vi "subDetermineNeedRebuildingFromHashes.vi"(8 "Force rebuild":bool, 9 "Dependency files":set{path}(c389), 10 "ProjectItem in":refnum<class "ProjectItem.lvclass">, 11 "Hashes in":T1) -> (1 "Needs rebuilding":bool, 2 "Log string":string, 3 "Hashes out":T1)   [LabVIEW 2019, in "SolutionBuilder.lvlib" / "SolutionBuilder.lvclass"]
uses:
  SolutionBuilder.lvclass
  Hashes.ctl
  HashMap.ctl
  IncrementalProjectInfo.ctl
  ProjectItem/ProjectItem.lvclass
  <vilib>/Utility/miscctls.llb/LVMapReplaceAction.ctl
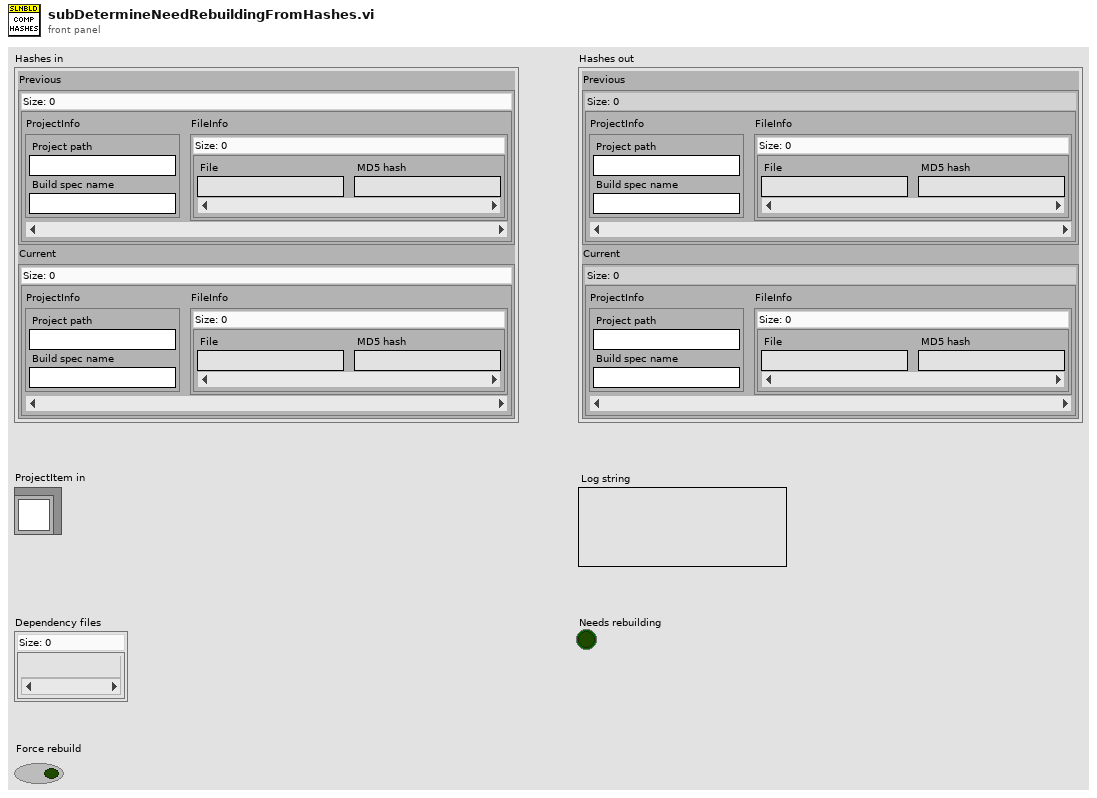
[diagram p1: front panel]
types:
  T1 = typedef "SolutionBuilder.lvlib/SolutionBuilder.lvclass/Hashes.ctl" = cluster{"Previous":T2, "Current":T2}
  T2 = typedef "SolutionBuilder.lvlib/SolutionBuilder.lvclass/HashMap.ctl" = map{T3, map{string, string}}
  T3 = typedef "SolutionBuilder.lvlib/SolutionBuilder.lvclass/IncrementalProjectInfo.ctl" = cluster{"Project path":string, "Build spec name":string}
  T4 = typedef "LVMapReplaceAction.ctl" = enum32{"Modify Entry only if found", "Add or Modify Entry", "Delete Entry"}
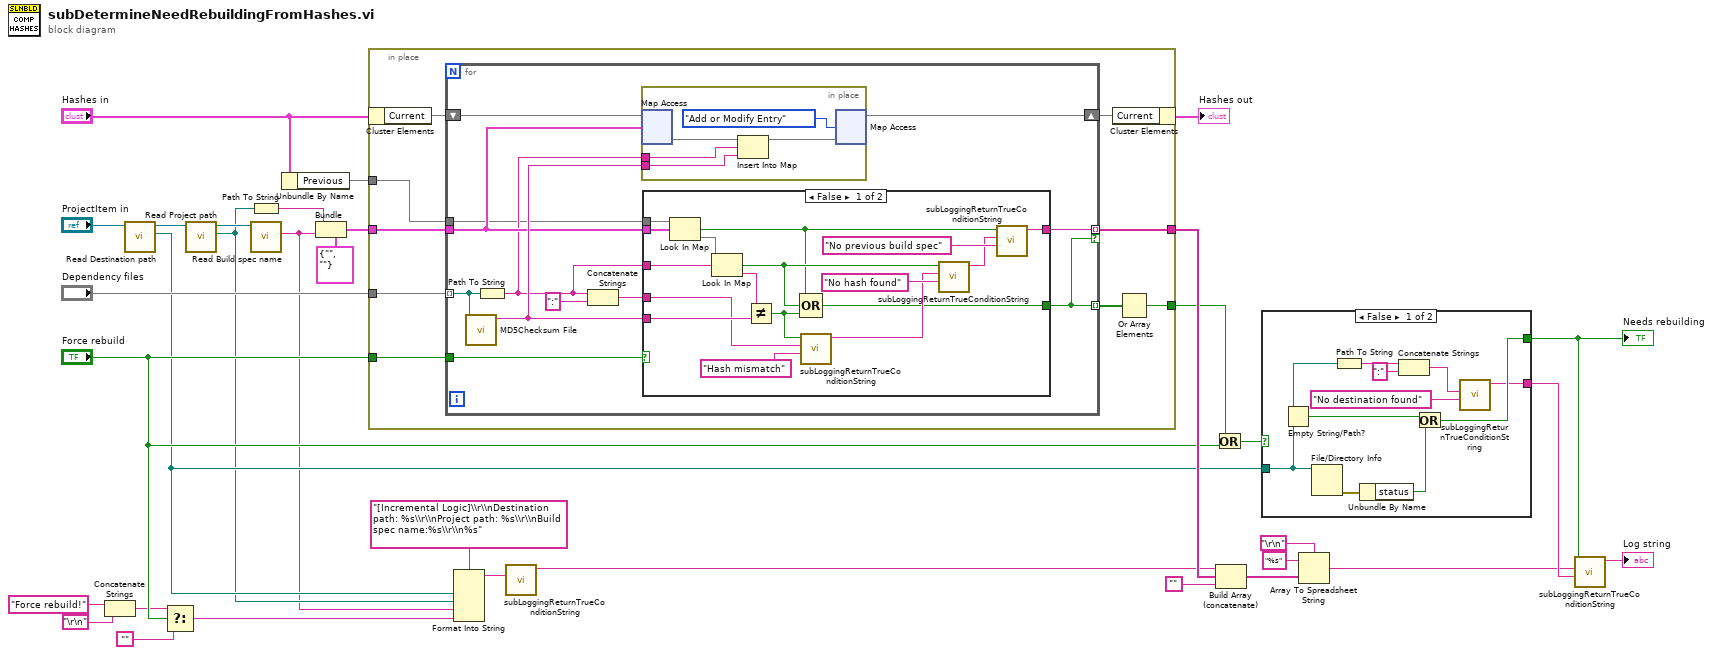
[diagram p0: block diagram]
diagram:
  n1 = Concatenate Strings("Force rebuild!" ("True string"), "\r\n") -> (w9:string)
  n2 = call-dynamic "Read Destination path.vi"("ProjectItem in"="ProjectItem in") -> ("Destination path"=w6:path, "ProjectItem out"=w27:refnum<class "ProjectItem.lvclass">)  [unwired: 9 in]
  n3 = Select(t=w9, s="Force rebuild", f="") -> (s? t:f=w3:string)
  n4 = call-dynamic "Read Project path.vi"("ProjectItem in"=w27) -> ("Project path"=w5:path, "ProjectItem out"=w26:refnum<class "ProjectItem.lvclass">)  [unwired: 9 in]
  n5 = Path To String(path=w5) -> (string=w29:string)
  n6 = call-dynamic "Read Build spec name.vi"("ProjectItem in"=w26) -> ("Build spec name"=w4:string)  [unwired: 9 in, 1 out]
  n7 = Unbundle By Name("Hashes in") -> ("Previous"=w15:T2)
  n8 = Bundle(cluster=T3 {"Project path"="", "Build spec name"=""} ("key"), "Project path"=w29, "Build spec name"=w4) -> (w28:T3)
  n9 = in-place {
    in-place-border: "Dependency files" -> [w42]
    in-place-border: w28 -> [w41]
    in-place-border: [w40] -> w23
    in-place-border: w15 -> [w37]
    in-place-border: "Force rebuild" -> [w36]
    in-place-border: [w34] -> w13
    n10 = in-place-cluster #1("Hashes in") -> ("Current"=w39:T2)
    n11 = for {
      shift-right: [w51] -> w38
      shift-left: w39 -> [w53]
      tunnel: w42 -> [w54] mode=indexing
      tunnel: [w45] -> w35 mode=indexing
      tunnel: w41 -> [w50]
      tunnel: [w46] -> w40 mode=indexing if=w45
      tunnel: w37 -> [w44]
      tunnel: w36 -> [w43]
      n12 = call <vilib>:"MD5Checksum File.vi"("Path"=w54) -> ("MD5 message-digest"=w52:string)  [unwired: 9 in, 1 out]
      n13 = Path To String(path=w54) -> (string=w49:string)
      n14 = Concatenate Strings(w49, ":" ("string")) -> (w47:string)
      n15 = in-place {
        in-place-border: w49 -> [w56]
        in-place-border: w52 -> [w55]
        n16 = in-place-map #2(w53, w50) -> (w59:map{string, string})  [unwired: 1 in, 1 out]
        n17 = Insert Into Map(map in=w59, key=w56, value=w55) -> (map out=w58:map{string, string})  [unwired: 2 out]
        n18 = in-place-map #2(w58, LVMapReplaceAction."Add or Modify Entry" ("action")) -> (w51:T2)  [unwired: 2 out]
      }
      n19 = case shown="False" w43 {
        tunnel: w44 -> [w76 _]
        tunnel: w52 -> [w73 _]
        tunnel: w50 -> [w72 _]
        tunnel: w49 -> [w65 _]
        tunnel: w47 -> [w64 _]
        tunnel: [w61 _] -> w46
        tunnel: [w60 _] -> w45
        frame False {
          n20 = Look In Map(map=w76, key=w72) -> (key not found?=w66:bool, value=w75:map{string, string})  [unwired: 1 in]
          n21 = Look In Map(map=w75, key=w65) -> (key not found?=w69:bool, value=w74:string)  [unwired: 1 in]
          n22 = Not Equal?(x=w74, y=w73) -> (x != y?=w70:bool)
          n23 = Compound Arithmetic op=OR(w66, w69, w70) -> (w60:bool)
          n24 = call "subLoggingReturnTrueConditionString.vi"("True string"="Hash mismatch" ("t"), "Initial string"=w64, "Condition (T)"=w70) -> ("Log string"=w63:string)  [unwired: 8 in]
          n25 = call "subLoggingReturnTrueConditionString.vi"("True string"="No hash found", "Initial string"=w63, "Condition (T)"=w69) -> ("Log string"=w62:string)  [unwired: 8 in]
          n26 = call "subLoggingReturnTrueConditionString.vi"("True string"="No previous build spec", "Initial string"=w62, "Condition (T)"=w66) -> ("Log string"=w61:string)  [unwired: 8 in]
        }
        frame True {
        }
      }
    }
    n27 = in-place-cluster #1("Current"=w38) -> (→"Hashes out":T1)
    n28 = Or Array Elements(Boolean array=w35) -> (logical OR=w34:bool)
  }
  n29 = Format Into String(format string="[Incremental Logic]\\r\\nDestination path: %s\\r\\nProject path: %s\\r\\nBuild spec name:%s\\r\\n%s", w6, w5, w4, w3) -> (resulting string=w2:string)  [unwired: 2 in, 1 out]
  n30 = call "subLoggingReturnTrueConditionString.vi"("Initial string"=w2) -> ("Log string"=w22:string)  [unwired: 10 in]
  n31 = Or(x=w13, y="Force rebuild") -> (x .or. y?=w12:bool)
  n32 = Build Array (concatenate)(w22, w23, "") -> (w21:string[])
  n33 = case shown="False" w12 {
    selector: w12 -> [_ w87]
    tunnel: [w83 w87] -> w17
    tunnel: w6 -> [w78 _]
    tunnel: [w81 _] -> w20
    frame False {
      n34 = Empty String/Path?(string/path=w78) -> (empty?=w85:bool)
      n35 = File/Directory Info(path=w78) -> (error out=w86:errorcluster)  [unwired: 1 in, 6 out]
      n36 = Path To String(path=w78) -> (string=w80:string)
      n37 = Unbundle By Name(w86) -> ("status"=w84:bool)
      n38 = Concatenate Strings(w80, ":" ("string")) -> (w77:string)
      n39 = Or(x=w85, y=w84) -> (x .or. y?=w83:bool)
      n40 = call "subLoggingReturnTrueConditionString.vi"("True string"="No destination found" ("String"), "Initial string"=w77) -> ("Log string"=w81:string)  [unwired: 9 in]
    }
    frame True {
    }
  }
  "Needs rebuilding" <- w17
  n41 = Array To Spreadsheet String(delimiter (Tab)="\r\n", array=w21, 3:"%s" ("format string")) -> (spreadsheet string=w19:string)
  n42 = call "subLoggingReturnTrueConditionString.vi"("True string"=w20, "Initial string"=w19, "Condition (T)"=w17) -> ("Log string"=→"Log string":string)  [unwired: 8 in]
